vi "Write Element of Guidance Array.vi"(8 "error in (no error)":errorcluster, 9 "Guidance Library.lvlib:Guidance.lvclass":refnum<class "Guidance.lvclass">, 10 "index":i32, 11 "Vessel in":refnum<class "Vessel.lvclass">) -> (0 "error out":errorcluster, 3 "Vessel out":refnum<class "Vessel.lvclass">)   [LabVIEW 2011, in "Vessel.lvclass"]
uses:
  Vessel.lvclass
  Guidance/Guidance.lvclass
  Vessel.lvclass/Vessel.ctl
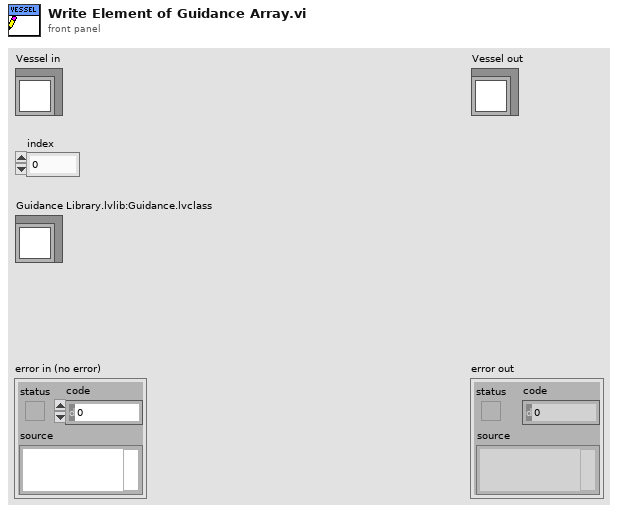
[diagram p1: front panel]
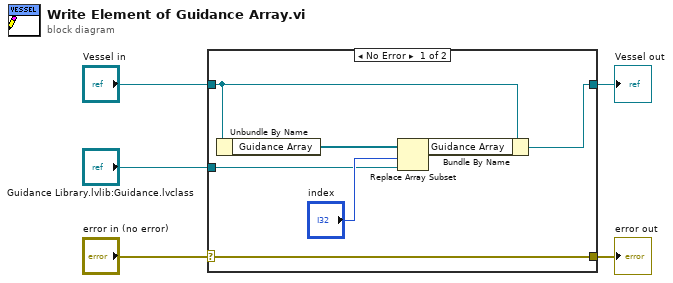
[diagram p0: block diagram]
diagram:
  n1 = case shown="No Error" "error in (no error)" {
    selector: "error in (no error)" -> [w12 w13]
    tunnel: [w12 w13] -> w4
    tunnel: [w11 w14] -> w2
    tunnel: "Vessel in" -> [w10 w14]
    tunnel: "Guidance Library.lvlib:Guidance.lvclass" -> [w6 _]
    frame No Error {
      n2 = Unbundle By Name(w10) -> ("Guidance Array"=w9:refnum<class "Guidance.lvclass">[])
      n3 = Replace Array Subset(array=w9, new element=w6, index="index") -> (w8:refnum<class "Guidance.lvclass">[])
      n4 = Bundle By Name(cluster=w10, "Guidance Array"=w8) -> (w11:refnum<class "Vessel.lvclass">)
    }
    frame Error {
    }
  }
  "error out" <- w4
  "Vessel out" <- w2
